vi "BuildModule (SubVI).vi"(0 "Module side length [mm]":dbl=97.54, 1 "Angle":dbl, 2 "Centre [mm]":cluster{"X":dbl, "Y":dbl, "Z":dbl}, 3 "x to fiducial [um]":dbl=230.0, 4 "y to fiducial [um]":dbl=1030.0, 5 "Units":enum16{"mrad", "Radians", "Degrees"}(ring)) -> (7 "Generated List of Module Coordinates":dbl[][](array[numeric]))   [LabVIEW 2016]
panel:
  out "y, centre":dbl
  out "x, centre":dbl
  out "Length":dbl
  out "A-B coordinates":cluster{"X":dbl, "Y":dbl, "Z":dbl}
  out "Created Module Graph":cluster{dbl[], dbl[]}(graph)
  out "A [mm]":cluster{"X":dbl, "Y":dbl, "Z":dbl}
  out "D [mm]":cluster{"X":dbl, "Y":dbl, "Z":dbl}
  out "C [mm]":cluster{"X":dbl, "Y":dbl, "Z":dbl}
  out "B [mm]":cluster{"X":dbl, "Y":dbl, "Z":dbl}
  out "lv [mm]":dbl
  out "lh [mm]":dbl
  # "BuildModule\n\nThis SubVI takes a centre coordinate and computes the positions of modules associated with that centre.\nThe SubVI also accepts a rotation angle to pivot the module."
  # "CROSS CHECKS"
  # "INPUTS"
  # "OUTPUTS"
  # "230 um for 4dots"
  # "230+300+500 um for 4dots"
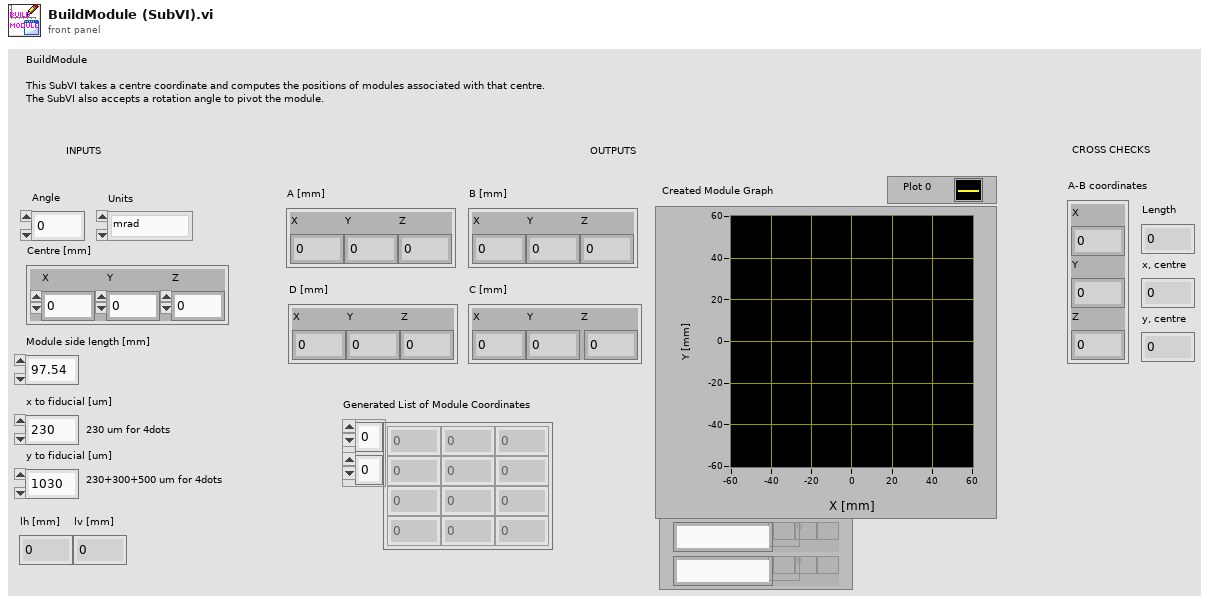
[diagram p1: front panel]
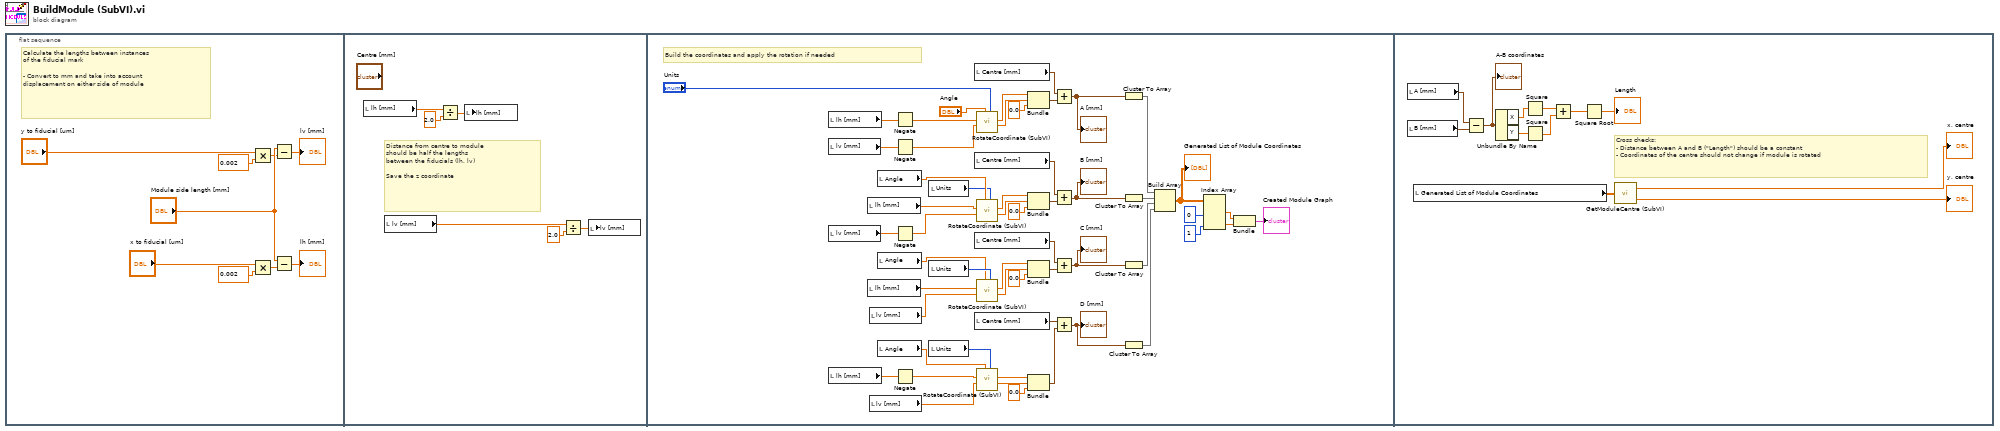
[diagram p0: block diagram]
diagram:
  n1 = flat-sequence {
    frame #0 {
      # "Calculate the lengths between instances\nof the fiducial mark\n\n- Convert to mm and take into account\ndisplacement on either side of module"
      n2 = Multiply(x="y to fiducial [um]", y=0.002) -> (x*y=w2:dbl)
      n3 = Multiply(x="x to fiducial [um]", y=0.002) -> (x*y=w5:dbl)
      n4 = Subtract(x="Module side length [mm]", y=w2) -> (x-y=→"lv [mm]":dbl)
      n5 = Subtract(x="Module side length [mm]", y=w5) -> (x-y=→"lh [mm]":dbl)
    }
    frame #1 {
      # "Distance from centre to module \nshould be half the lengths\nbetween the fiducials (lh, lv)\n\nSave the z coordinate"
      n6 = local read "lh [mm]"() -> (w10:dbl)
      n7 = local read "lv [mm]"() -> (w15:dbl)
      n8 = Divide(x=w10, y=2.0) -> (x/y=w12:dbl)
      n9 = local write "lh [mm]"(w12) -> ()
      n10 = Divide(x=w15, y=2.0) -> (x/y=w13:dbl)
      n11 = local write "lv [mm]"(w13) -> ()
    }
    frame #2 {
      # "Build the coordinates and apply the rotation if needed"
      n12 = local read "lh [mm]"() -> (w56:dbl)
      n13 = local read "lv [mm]"() -> (w55:dbl)
      n14 = local read "lv [mm]"() -> (w52:dbl)
      n15 = local read "lh [mm]"() -> (w50:dbl)
      n16 = local read "lh [mm]"() -> (w25:dbl)
      n17 = local read "lh [mm]"() -> (w29:dbl)
      n18 = local read "lv [mm]"() -> (w28:dbl)
      n19 = local read "lv [mm]"() -> (w23:dbl)
      n20 = local read "Angle"() -> (w58:dbl)
      n21 = local read "Angle"() -> (w59:dbl)
      n22 = local read "Angle"() -> (w51:dbl)
      n23 = Negate(x=w56) -> (-x=w17:dbl)
      n24 = Negate(x=w55) -> (-x=w16:dbl)
      n25 = Negate(x=w52) -> (-x=w24:dbl)
      n26 = Negate(x=w50) -> (-x=w22:dbl)
      n27 = local read "Units"() -> (w57:enum16{"mrad", "Radians", "Degrees"})
      n28 = local read "Units"() -> (w60:enum16{"mrad", "Radians", "Degrees"})
      n29 = local read "Units"() -> (w61:enum16{"mrad", "Radians", "Degrees"})
      n30 = local read "Centre [mm]"() -> (w40:cluster{"X":dbl, "Y":dbl, "Z":dbl})
      n31 = local read "Centre [mm]"() -> (w46:cluster{"X":dbl, "Y":dbl, "Z":dbl})
      n32 = local read "Centre [mm]"() -> (w44:cluster{"X":dbl, "Y":dbl, "Z":dbl})
      n33 = local read "Centre [mm]"() -> (w42:cluster{"X":dbl, "Y":dbl, "Z":dbl})
      n34 = call "RotateCoordinate (SubVI).vi"("Units"="Units", "Angle"="Angle", "y"=w16, "x"=w17) -> ("y'"=w30:dbl, "x'"=w31:dbl)  [unwired: 5 in, 1 out]
      n35 = call "RotateCoordinate (SubVI).vi"("Units"=w57, "Angle"=w58, "y"=w24, "x"=w25) -> ("y'"=w26:dbl, "x'"=w27:dbl)  [unwired: 5 in, 1 out]
      n36 = call "RotateCoordinate (SubVI).vi"("Units"=w60, "Angle"=w59, "y"=w28, "x"=w29) -> ("y'"=w34:dbl, "x'"=w35:dbl)  [unwired: 5 in, 1 out]
      n37 = call "RotateCoordinate (SubVI).vi"("Units"=w61, "Angle"=w51, "y"=w23, "x"=w22) -> ("y'"=w20:dbl, "x'"=w21:dbl)  [unwired: 5 in, 1 out]
      n38 = Bundle("x'"=w31, "y'"=w30, "y"=0.0) -> (w32:cluster{"x'":dbl, "y'":dbl, "y":dbl})  [unwired: 1 in]
      n39 = Bundle("x'"=w27, "y'"=w26, "y"=0.0) -> (w18:cluster{"x'":dbl, "y'":dbl, "y":dbl})  [unwired: 1 in]
      n40 = Bundle("x'"=w35, "y'"=w34, "y"=0.0) -> (w33:cluster{"x'":dbl, "y'":dbl, "y":dbl})  [unwired: 1 in]
      n41 = Bundle("x'"=w21, "y'"=w20, "y"=0.0) -> (w19:cluster{"x'":dbl, "y'":dbl, "y":dbl})  [unwired: 1 in]
      n42 = Add(x=w40, y=w32) -> (x+y=w47:cluster{dbl, dbl, dbl})
      "A [mm]" <- w47
      n43 = Add(x=w46, y=w18) -> (x+y=w45:cluster{dbl, dbl, dbl})
      "B [mm]" <- w45
      n44 = Add(x=w44, y=w33) -> (x+y=w43:cluster{dbl, dbl, dbl})
      "C [mm]" <- w43
      n45 = Add(x=w42, y=w19) -> (x+y=w41:cluster{dbl, dbl, dbl})
      "D [mm]" <- w41
      n46 = Cluster To Array(cluster=w47) -> (array=w62:dbl[])
      n47 = Cluster To Array(cluster=w45) -> (array=w63:dbl[])
      n48 = Cluster To Array(cluster=w43) -> (array=w64:dbl[])
      n49 = Cluster To Array(cluster=w41) -> (array=w65:dbl[])
      n50 = Build Array(w62, w63, w64, w65) -> (w49:dbl[][])
      "Generated List of Module Coordinates" <- w49
      n51 = Index Array(array=w49, index (col) #1=0 ("disabled index (col)"), index (col) #2=1 ("index (col)")) -> (element #1=w68:dbl[], element #2=w69:dbl[])  [unwired: 2 in]
      n52 = Bundle(w68, w69) -> (→"Created Module Graph":cluster{dbl[], dbl[]})  [unwired: 1 in]
    }
    frame #3 {
      # "Cross checks: \n- Distance between A and B (\"Length\") should be a constant\n- Coordinates of the centre should not change if module is rotated"
      n53 = local read "A [mm]"() -> (w81:cluster{"X":dbl, "Y":dbl, "Z":dbl})
      n54 = local read "B [mm]"() -> (w80:cluster{"X":dbl, "Y":dbl, "Z":dbl})
      n55 = local read "Generated List of Module Coordinates"() -> (w72:dbl[][])
      n56 = Subtract(x=w81, y=w80) -> (x-y=w79:cluster{"X":dbl, "Y":dbl, "Z":dbl})
      "A-B coordinates" <- w79
      n57 = Unbundle By Name(w79) -> ("X"=w78:dbl, "Y"=w77:dbl)
      n58 = Square(x=w78) -> (x^2=w76:dbl)
      n59 = Square(x=w77) -> (x^2=w75:dbl)
      n60 = Add(x=w76, y=w75) -> (x+y=w74:dbl)
      n61 = Square Root(x=w74) -> (sqrt(x)=→"Length":dbl)
      n62 = call "GetModuleCentre (SubVI).vi"("4x3 Array of Fiducial Coordinates"=w72) -> ("x, centre"=→"x, centre":dbl, "y, centre"=→"y, centre":dbl)
    }
  }
